vi "vision logic.vi"() -> ()   [LabVIEW 2018]
uses:
  <vilib>/Rock Robotics/Network Tables/NT Read Number.vi
  <vilib>/Rock Robotics/Network Tables/NT Read Boolean.vi
  <vilib>/Rock Robotics/Network Tables/NT Write Number.vi
  <vilib>/Rock Robotics/WPI/Utilities/WPI_GetSetVariantRefNum.vi
  <vilib>/Rock Robotics/Network Tables/NT Write Numeric Array.vi
  <vilib>/Rock Robotics/Network Tables/NT Write Boolean.vi
panel:
  out "RobotDrive Motors":dbl
  in  "Tab Control":T1(tab)
  in  "High Threshold":dbl=1.8
  in  "Low Threshold":dbl=1.2
  out "Center of Centroid":dbl
  out "Sonar1 Value":dbl
  in  "Wall (Sonar)":dbl=3.0
  in  "LX axis":dbl=0.7000000000000001 min=-1.0 max=1.0 step=0.05
  in  "LY axis":dbl=-0.6 min=-1.0 max=1.0 step=0.05
  in  "RX axis":dbl=0.6 min=-1.0 max=1.0 step=0.05
  in  "RY axis":dbl=-0.7500000000000001 min=-1.0 max=1.0 step=0.05
  in  "X axis":dbl=0.7000000000000001 min=-1.0 max=1.0 step=0.05
  in  "Y axis":dbl=-0.7000000000000001 min=-1.0 max=1.0 step=0.05
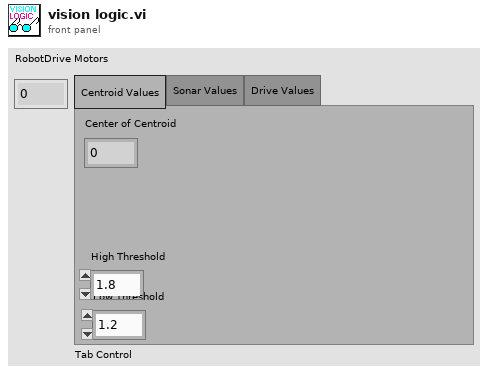
[diagram p1: front panel]
types:
  T1 = enum32{"Centroid Values", "Sonar Values", "Drive Values"}
  T2 = typedef "WPI_RobotDriveDevRef.ctl" = cluster{"DevStatus":errorcluster, "Motors[]":T3[], "Square Inputs":bool, "Max Output":dbl}
  T3 = typedef "WPI_MotorControlDeviceRef.ctl" = cluster{"DeviceStatus":errorcluster, "Type":T4, "PWM":cluster{"PWM Channel":T5, "DeadBand":T6}, "CAN":cluster{"Device Number":u8, "SetOutput VI Ref":variant, "GetOutput VI Ref":variant, "Enable VI Ref":variant, "Disable VI Ref":variant, "Data":variant}, "Invert":bool, "DIO PWM":cluster{"PWM \"Enable\" Channel":T5, "DIOChannel":T7, "PWM Rate":dbl}}
  T4 = typedef "WPI_MotorControlType.ctl" = enum16{"PWM", "CAN", "DIO PWM"}
  T5 = typedef "FPGA_DIOPWMChannel.ctl" = enum8{"PWM 0", "PWM 1", "PWM 2", "PWM 3", "PWM 4", "PWM 5", "PWM 6", "PWM 7", "PWM 8", "PWM 9", "PWM MXP 0", "PWM MXP 1", "PWM MXP 2", "PWM MXP 3", "PWM MXP 4", "PWM MXP 5", "PWM MXP 6", "PWM MXP 7", "PWM MXP 8", "PWM MXP 9", "Invalid"}
  T6 = typedef "WPI_PWMDeadband.ctl" = cluster{"Name":string, "maxPositivePwm":i32, "minPositivePwm":i32, "centerPwm":i32, "maxNegativePwm":i32, "minNegativePwm":i32, "angularRange":u16}
  T7 = typedef "FPGA_DIOChannel.ctl" = enum8{"DIO 0", "DIO 1", "DIO 2", "DIO 3", "DIO 4", "DIO 5", "DIO 6", "DIO 7", "DIO 8", "DIO 9", "DIO MXP 0", "DIO MXP 1", "DIO MXP 2", "DIO MXP 3", "DIO MXP 4", "DIO MXP 5", "DIO MXP 6", "DIO MXP 7", "DIO MXP 8", "DIO MXP 9", "DIO MXP 10", "DIO MXP 11", "DIO MXP 12", "DIO MXP 13", "DIO MXP 14", "DIO MXP 15", "SPI Port CS1", "SPI Port CS2", "SPI Port CS3", "SPI Port MISO", "SPI Port MOSI", "Invalid"}
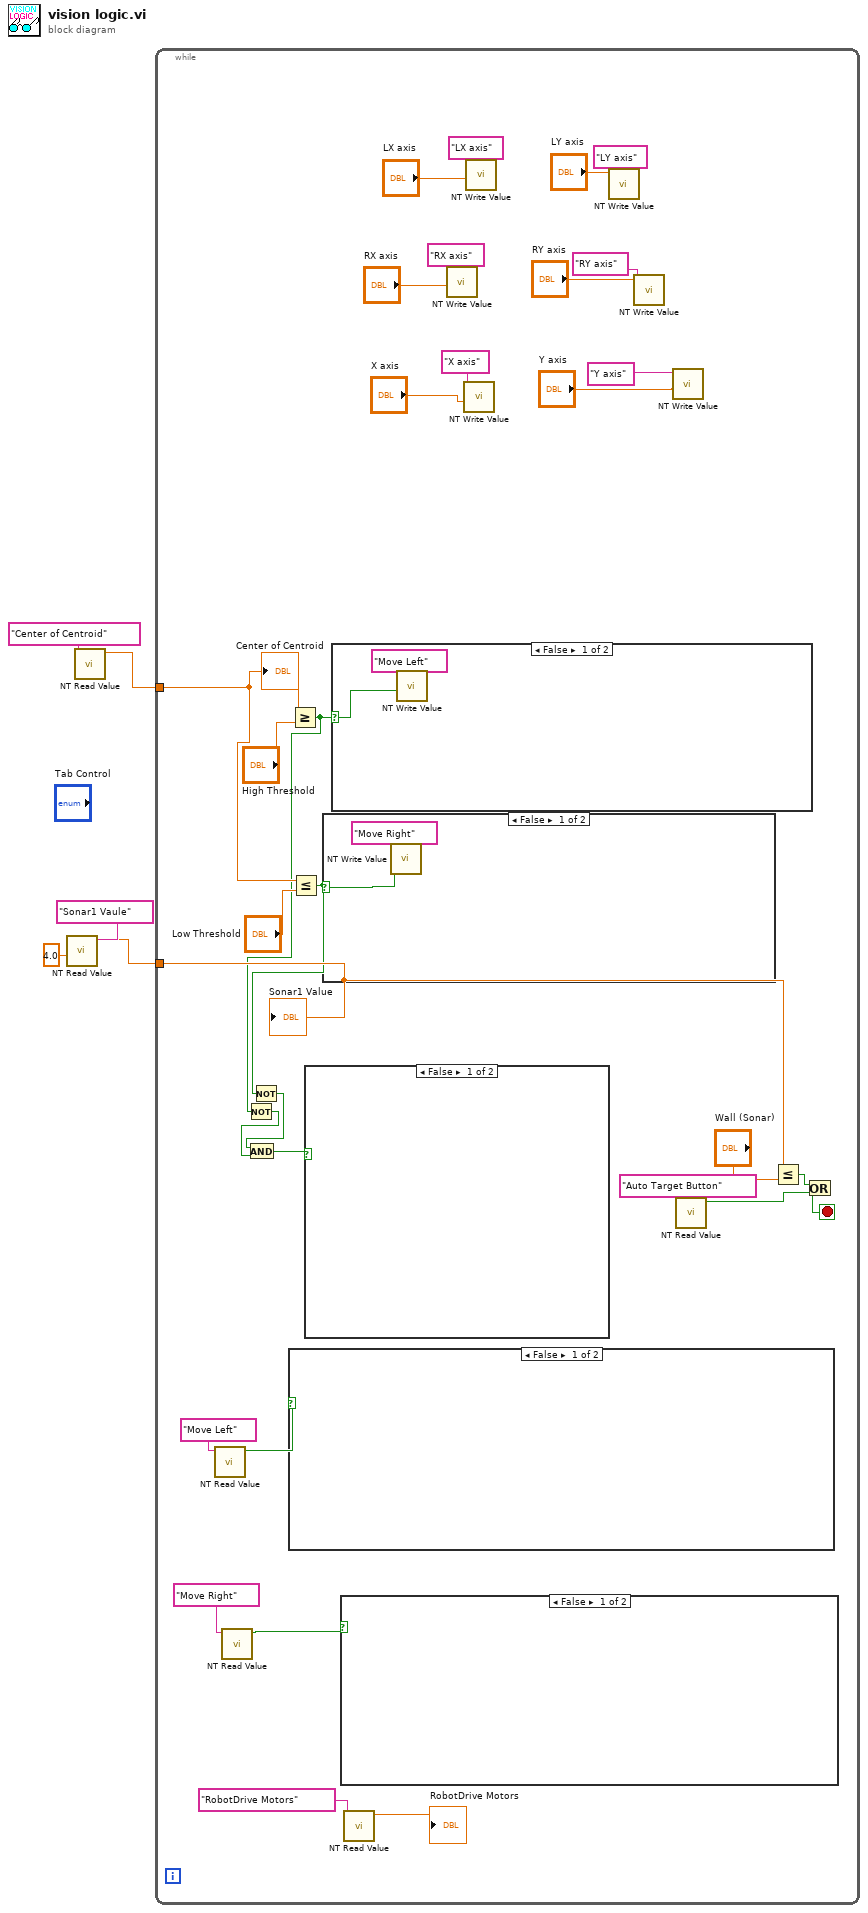
[diagram p0: block diagram]
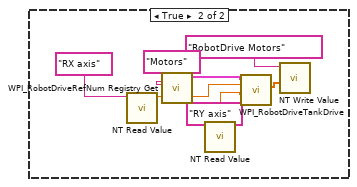
[diagram p2: hidden frame]
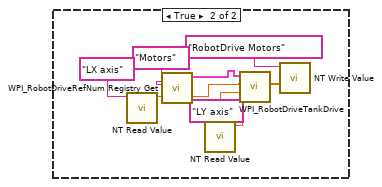
[diagram p3: hidden frame]
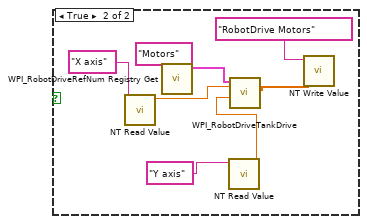
[diagram p4: hidden frame]
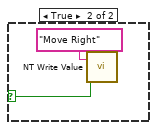
[diagram p5: hidden frame]
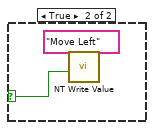
[diagram p6: hidden frame]
diagram:
  n1 = call-poly <vilib>:"NT Read Value.vi"("Default Value"=4.0, "Name"="Sonar1 Vaule") -> ("Numeric"=w4:dbl)  [unwired: 8 in, 1 out]
  n2 = call-poly <vilib>:"NT Read Value.vi"("Name"="Center of Centroid") -> ("Numeric"=w2:dbl)  [unwired: 9 in, 1 out]
  n3 = while {
    tunnel: w4 -> [w30]
    tunnel: w2 -> [w32]
    stop <- w37 stop-if-true
    n4 = call-poly <vilib>:"NT Read Value.vi"("Name"="Move Left") -> ("Boolean"=w23:bool)  [unwired: 9 in, 1 out]
    n5 = call-poly <vilib>:"NT Read Value.vi"("Name"="Move Right") -> ("Boolean"=w21:bool)  [unwired: 9 in, 1 out]
    n6 = case shown="False" w23 {
      frame False {
      }
      frame True {
        n7 = call-poly <vilib>:"NT Read Value.vi"("Name"="LX axis") -> ("Numeric"=w47:dbl)  [unwired: 9 in, 1 out]
        n8 = call <vilib>:"WPI_RobotDriveRefNum Registry Get.vi"("refnum name"="Motors") -> ("RobotDriveDevRef"=w48:T2)  [unwired: 1 in, 9 out]
        n9 = call-poly <vilib>:"NT Read Value.vi"("Name"="LY axis") -> ("Numeric"=w46:dbl)  [unwired: 9 in, 1 out]
        n10 = call <vilib>:"WPI_RobotDriveTankDrive.vi"("Right axis value"=w46, "Left axis value"=w47, "RobotDriveDevRef"=w48) -> ("Motor Values"=w49:dbl[])  [unwired: 6 in, 2 out]
        n11 = call-poly <vilib>:"NT Write Value.vi"("Numeric Array"=w49, "Name"="RobotDrive Motors") -> ()  [unwired: 9 in, 1 out]
      }
    }
    n12 = Greater Or Equal?(x=w32, y="High Threshold") -> (x >= y?=w26:bool)
    n13 = Not(x=w26) -> (.not. x?=w25:bool)
    n14 = Less Or Equal?(x=w32, y="Low Threshold") -> (x <= y?=w28:bool)
    n15 = Not(x=w28) -> (.not. x?=w27:bool)
    n16 = And(x=w27, y=w25) -> (x .and. y?=w24:bool)
    n17 = case shown="False" w24 {
      frame False {
      }
      frame True {
        n18 = call-poly <vilib>:"NT Read Value.vi"("Name"="X axis") -> ("Numeric"=w56:dbl)  [unwired: 9 in, 1 out]
        n19 = call <vilib>:"WPI_RobotDriveRefNum Registry Get.vi"("refnum name"="Motors") -> ("RobotDriveDevRef"=w54:T2)  [unwired: 1 in, 9 out]
        n20 = call-poly <vilib>:"NT Read Value.vi"("Name"="Y axis") -> ("Numeric"=w55:dbl)  [unwired: 9 in, 1 out]
        n21 = call <vilib>:"WPI_RobotDriveTankDrive.vi"("Right axis value"=w55, "Left axis value"=w56, "RobotDriveDevRef"=w54) -> ("Motor Values"=w57:dbl[])  [unwired: 6 in, 2 out]
        n22 = call-poly <vilib>:"NT Write Value.vi"("Numeric Array"=w57, "Name"="RobotDrive Motors") -> ()  [unwired: 9 in, 1 out]
      }
    }
    n23 = case shown="False" w28 {
      selector: w28 -> [w62 w65]
      frame False {
        n24 = call-poly <vilib>:"NT Write Value.vi"("Boolean"=w62, "Name"="Move Right") -> ()  [unwired: 9 in, 1 out]
      }
      frame True {
        n25 = call-poly <vilib>:"NT Write Value.vi"("Boolean"=w65, "Name"="Move Right") -> ()  [unwired: 9 in, 1 out]
      }
    }
    n26 = case shown="False" w26 {
      selector: w26 -> [w66 w69]
      frame False {
        n27 = call-poly <vilib>:"NT Write Value.vi"("Boolean"=w66, "Name"="Move Left") -> ()  [unwired: 9 in, 1 out]
      }
      frame True {
        n28 = call-poly <vilib>:"NT Write Value.vi"("Boolean"=w69, "Name"="Move Left") -> ()  [unwired: 9 in, 1 out]
      }
    }
    n29 = case shown="False" w21 {
      frame False {
      }
      frame True {
        n30 = call-poly <vilib>:"NT Read Value.vi"("Name"="RX axis") -> ("Numeric"=w39:dbl)  [unwired: 9 in, 1 out]
        n31 = call <vilib>:"WPI_RobotDriveRefNum Registry Get.vi"("refnum name"="Motors") -> ("RobotDriveDevRef"=w40:T2)  [unwired: 1 in, 9 out]
        n32 = call-poly <vilib>:"NT Read Value.vi"("Name"="RY axis") -> ("Numeric"=w38:dbl)  [unwired: 9 in, 1 out]
        n33 = call <vilib>:"WPI_RobotDriveTankDrive.vi"("Right axis value"=w38, "Left axis value"=w39, "RobotDriveDevRef"=w40) -> ("Motor Values"=w41:dbl[])  [unwired: 6 in, 2 out]
        n34 = call-poly <vilib>:"NT Write Value.vi"("Numeric Array"=w41, "Name"="RobotDrive Motors") -> ()  [unwired: 9 in, 1 out]
      }
    }
    n35 = call-poly <vilib>:"NT Read Value.vi"("Name"="RobotDrive Motors") -> ("Numeric"=→"RobotDrive Motors":dbl)  [unwired: 9 in, 1 out]
    n36 = call-poly <vilib>:"NT Write Value.vi"("Numeric"="RX axis", "Name"="RX axis") -> ()  [unwired: 9 in, 1 out]
    n37 = call-poly <vilib>:"NT Write Value.vi"("Numeric"="X axis", "Name"="X axis") -> ()  [unwired: 9 in, 1 out]
    n38 = call-poly <vilib>:"NT Write Value.vi"("Numeric"="LX axis", "Name"="LX axis") -> ()  [unwired: 9 in, 1 out]
    n39 = call-poly <vilib>:"NT Write Value.vi"("Numeric"="LY axis", "Name"="LY axis") -> ()  [unwired: 9 in, 1 out]
    n40 = call-poly <vilib>:"NT Write Value.vi"("Numeric"="RY axis", "Name"="RY axis") -> ()  [unwired: 9 in, 1 out]
    n41 = call-poly <vilib>:"NT Write Value.vi"("Numeric"="Y axis", "Name"="Y axis") -> ()  [unwired: 9 in, 1 out]
    n42 = call-poly <vilib>:"NT Read Value.vi"("Name"="Auto Target Button") -> ("Boolean"=w36:bool)  [unwired: 9 in, 1 out]
    n43 = Less Or Equal?(x=w30, y="Wall (Sonar)") -> (x <= y?=w34:bool)
    n44 = Or(x=w34, y=w36) -> (x .or. y?=w37:bool)
    "Sonar1 Value" <- w30
    "Center of Centroid" <- w32
  }
